vi "Auto Loop 4.vi"(10 "auto #":u32, 11 "Call Context":T1) -> (0 "Loop 4 Value2":dbl, 1 "Loop 4 Value1":dbl, 2 "Loop 4 exit value":i32, 3 "Loop 4 SubState":T2=enum."auto")   [LabVIEW 2011]
uses:
  subStates.ctl
  <vilib>/Rock Robotics/WPI/DriverStation/WPI_DriverStationDerivedRobotMode.ctl
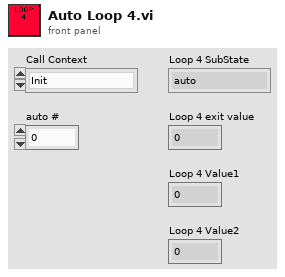
[diagram p1: front panel]
types:
  T1 = typedef "WPI_DriverStationDerivedRobotMode.ctl" = enum16{"Init", "Execute", "Stop"}
  T2 = typedef "subStates.ctl" = enum16{"null", "wait", "driver control", "auto", "manual override", "autoDrive", "hold position", "rotate", "end"}
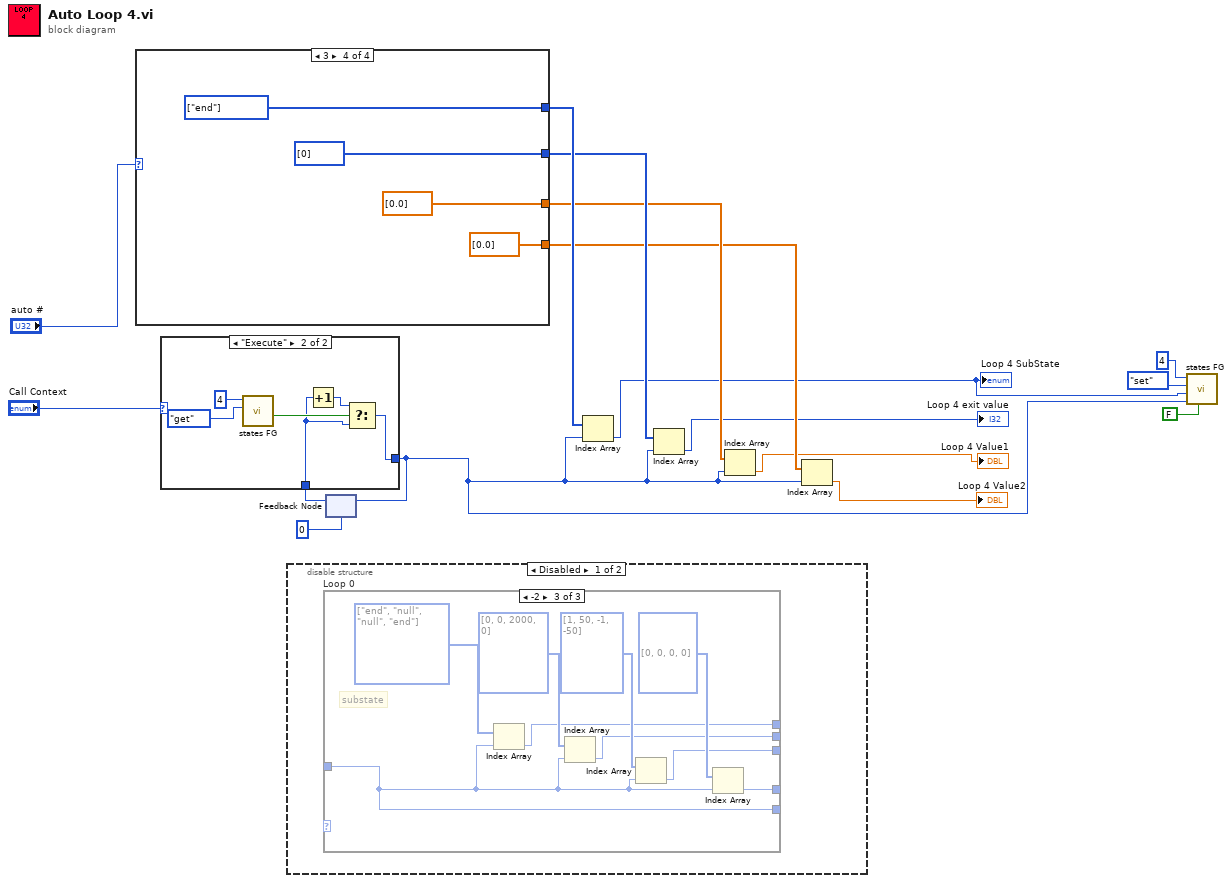
[diagram p0: block diagram]
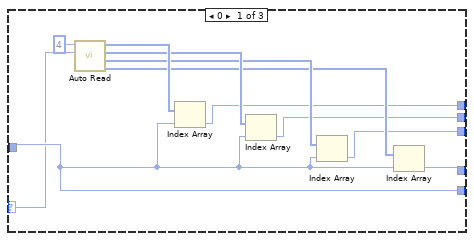
[diagram p2: hidden frame]
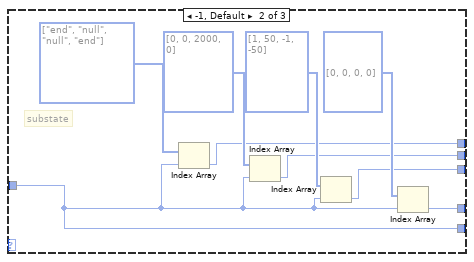
[diagram p3: hidden frame]
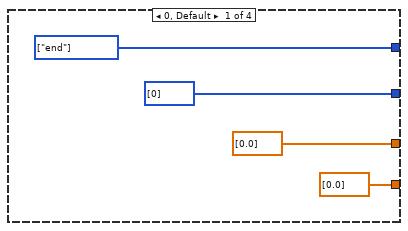
[diagram p5: hidden frame]
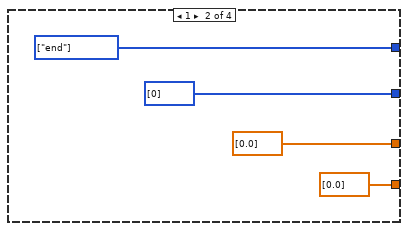
[diagram p6: hidden frame]
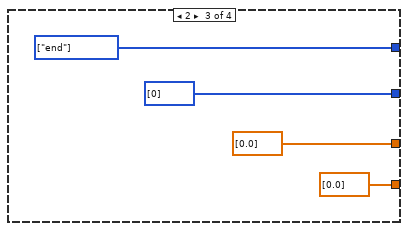
[diagram p7: hidden frame]
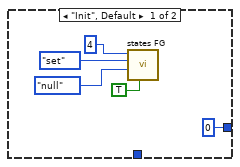
[diagram p8: hidden frame]
diagram:
  n1 = case shown="3" "auto #" {
    tunnel: [dbl[] [0.0] ("value2 array") dbl[] [0.0] ("value2 array") dbl[] [0.0] ("value2 array") dbl[] [0.0] ("value2 array")] -> w8
    tunnel: [dbl[] [0.0] ("value1 array") dbl[] [0.0] ("value1 array") dbl[] [0.0] ("value1 array") dbl[] [0.0] ("value1 array")] -> w9
    tunnel: [w18 w22 w26 w30] -> w11
    tunnel: [i32[] [0] ("exit value array") i32[] [0] ("exit value array") i32[] [0] ("exit value array") i32[] [0] ("exit value array")] -> w10
    frame 0, Default {
      w18 = T2[] [enum."end"] items=["null", "wait", "driver control", "auto", "manual override", "autoDrive", "hold position", "rotate", "end"] ("substate array")
    }
    frame 1 {
      w22 = T2[] [enum."end"] items=["null", "wait", "driver control", "auto", "manual override", "autoDrive", "hold position", "rotate", "end"] ("substate array")
    }
    frame 2 {
      w26 = T2[] [enum."end"] items=["null", "wait", "driver control", "auto", "manual override", "autoDrive", "hold position", "rotate", "end"] ("substate array")
    }
    frame 3 {
      w30 = T2[] [enum."end"] items=["null", "wait", "driver control", "auto", "manual override", "autoDrive", "hold position", "rotate", "end"] ("substate array")
    }
  }
  n2 = disable-structure shown="Disabled" {
    frame Disabled {
      n3 = case "Loop 0" shown="-2" {
        selector: _ -> [w33 _ _]
        tunnel: _ -> [w42 w44 w53]
        tunnel: [w37 w48 w57] -> _
        tunnel: [w36 w47 w56] -> _
        tunnel: [w35 w46 w55] -> _
        tunnel: [w34 w45 w54] -> _
        tunnel: [w42 w44 w53] -> _
        frame 0 {
          n4 = call "Auto Read.vi"("auto#"=w33, "loop #"=4) -> ("value 2s"=w38:i32[], "value 1s"=w39:i32[], "exit values"=w40:i32[], "substates"=w41:T2[])  [unwired: 6 in]
          n5 = Index Array(array=w41, index=w42) -> (element=w37:T2)
          n6 = Index Array(array=w40, index=w42) -> (element=w36:i32)
          n7 = Index Array(array=w39, index=w42) -> (element=w35:i32)
          n8 = Index Array(array=w38, index=w42) -> (element=w34:i32)
        }
        frame -1, Default {
          w52 = T2[] [enum."end", enum."null", enum."null", enum."end"] items=["null", "wait", "driver control", "auto", "manual override", "autoDrive", "hold position", "rotate", "end"] ("SubState Array")
          # "val2"
          # "val1"
          # "exit"
          # "substate"
          n9 = Index Array(array=w52, index=w44) -> (element=w48:T2)
          n10 = Index Array(array=i32[] [0, 0, 2000, 0], index=w44) -> (element=w47:i32)
          n11 = Index Array(array=i32[] [1, 50, -1, -50], index=w44) -> (element=w46:i32)
          n12 = Index Array(array=i32[] [0, 0, 0, 0], index=w44) -> (element=w45:i32)
        }
        frame -2 {
          w61 = T2[] [enum."end", enum."null", enum."null", enum."end"] items=["null", "wait", "driver control", "auto", "manual override", "autoDrive", "hold position", "rotate", "end"] ("SubState Array")
          # "val2"
          # "val1"
          # "exit"
          # "substate"
          n13 = Index Array(array=w61, index=w53) -> (element=w57:T2)
          n14 = Index Array(array=i32[] [0, 0, 2000, 0], index=w53) -> (element=w56:i32)
          n15 = Index Array(array=i32[] [1, 50, -1, -50], index=w53) -> (element=w55:i32)
          n16 = Index Array(array=i32[] [0, 0, 0, 0], index=w53) -> (element=w54:i32)
        }
      }
    }
    frame Enabled {
    }
  }
  n17 = feedback #1(0 ("Value1 2")) -> (w13:i32)
  n18 = case shown="\"Execute\"" "Call Context" {
    tunnel: [0 ("Value1 2") w71] -> w2
    tunnel: w13 -> [_ w68]
    frame "Init", Default {
      n19 = call "states FG.vi"("exit in"=TRUE, "subState in"=subStates."null", "menu (get)"=enum16{"set", "get"}."set", "Loop ID"=4) -> ()  [unwired: 4 in, 4 out]
    }
    frame "Execute" {
      n20 = call "states FG.vi"("menu (get)"=enum16{"set", "get"}."get", "Loop ID"=4) -> ("exit out"=w70:bool)  [unwired: 6 in, 3 out]
      n21 = Increment(x=w68) -> (x+1=w72:i32)
      n22 = Select(t=w72, s=w70, f=w68) -> (s? t:f=w71:i32)
    }
  }
  n23 = feedback-in #1(w2) -> ()
  n24 = Index Array(array=w11, index=w2) -> (element=w1:T2)
  "Loop 4 SubState" <- w1
  n25 = Index Array(array=w10, index=w2) -> (element=→"Loop 4 exit value":i32)
  n26 = Index Array(array=w9, index=w2) -> (element=→"Loop 4 Value1":dbl)
  n27 = Index Array(array=w8, index=w2) -> (element=→"Loop 4 Value2":dbl)
  n28 = call "states FG.vi"("exit in"=FALSE, "state # in"=w2, "subState in"=w1, "menu (get)"=enum16{"set", "get"}."set", "Loop ID"=4) -> ()  [unwired: 3 in, 4 out]
